vi "ifr2025 Protection.vi"(7 "Stop (0)":i16 format="%.0g", 8 "error in (no error)":errorcluster {"code" format="%.0x"}, 9 "Start (0)":i16 format="%.0g", 10 "State (Off)":bool, 11 "instrument handle":refnum<visa-resource-name>) -> (0 "error out":errorcluster {"code" format="%.0x"}, 3 "instrument handle out":refnum<visa-resource-name>)   [LabVIEW 2009]
doc: "This command specifies either a single location or a block of locations to be write-protected.\n\nAny protection applied to RAM will be lost on power down."
uses:
  Ifr2025_32.dll
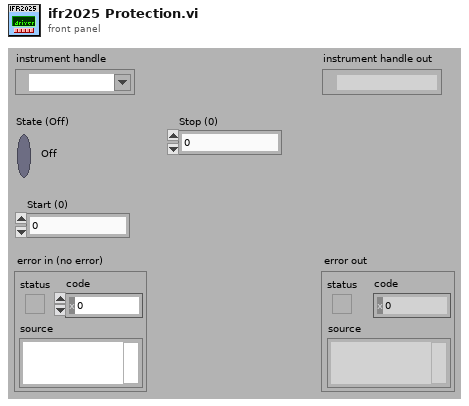
[diagram p1: front panel]
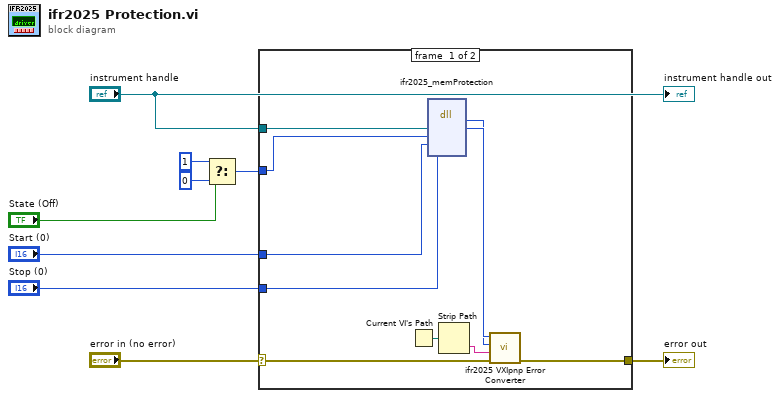
[diagram p0: block diagram]
diagram:
  n1 = Select(t=u16 1, s="State (Off)", f=u16 0) -> (s? t:f=w3:u16)
  n2 = case shown="No Error" "error in (no error)" {
    selector: "error in (no error)" -> [w14 w20]
    tunnel: [w13 w20] -> w9
    tunnel: "instrument handle" -> [w18 _]
    tunnel: w3 -> [w12 _]
    tunnel: "Start (0)" -> [w11 _]
    tunnel: "Stop (0)" -> [w10 _]
    frame #0 {
      n3 = Current VI's Path() -> (path=w19:path)
      n4 = dll-call lib="P:/inst/Marconi 2024 Signal Generator/source/labview/ifr2025/ifr2025/ifr2025_*.*" fn="ifr2025_memProtection"("vi"=w18, "State"=w12, "Start"=w11, "Stop"=w10) -> (w16:i32, "vi"=w17:u32)  [unwired: 6 in, 2 out]
      n5 = Strip Path(path=w19) -> (name=w15:string)  [unwired: 1 out]
      n6 = call "ifr2025 VXIpnp Error Converter.vi"("error in (no error)"=w14, "name of VI (\"\")"=w15, "CVI error code (0)"=w16, "instrument handle"=w17) -> ("error out"=w13:errorcluster)  [unwired: 7 out]
    }
    frame #1 {
    }
  }
  "error out" <- w9
  "instrument handle out" <- "instrument handle"
